vi "sendOpenLog.vi"(8 "error in (no error)":errorcluster, 11 "source":string) -> (0 "error out":errorcluster)   [LabVIEW 2017, in "loggingModule.lvlib"]
uses:
  loggingModule.lvlib
  Queue/TypeDefs/queueFGVState.ctl
  Queue/TypeDefs/message.ctl
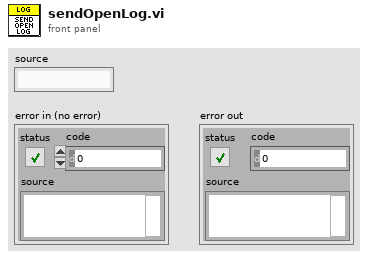
[diagram p1: front panel]
types:
  T1 = typedef "loggingModule.lvlib/message.ctl" = cluster{"calling module":string, "message":string, "data":variant}
  T2 = typedef "loggingModule.lvlib/queueFGVState.ctl" = enum16{"obtain", "enqueue low priority", "enqueue high priority", "dequeue", "release"}
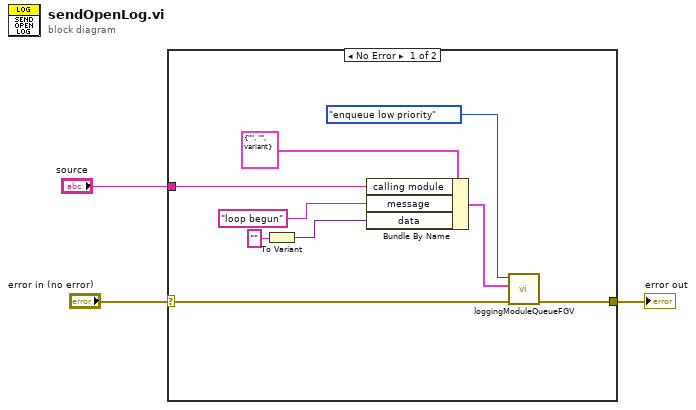
[diagram p0: block diagram]
diagram:
  n1 = case shown="No Error" "error in (no error)" {
    selector: "error in (no error)" -> [w4 w13]
    tunnel: [w12 w13] -> w3
    tunnel: "source" -> [w7 _]
    frame No Error {
      n2 = To Variant(anything="") -> (Variant=w10:variant)
      n3 = Bundle By Name(cluster=T1 {"calling module"="", "message"="", "data"=variant} ("message in"), "calling module"=w7, "message"="loop begun", "data"=w10) -> (w11:T1)
      n4 = call "loggingModuleQueueFGV.vi"("error in (no error)"=w4, "message in"=w11, "command"=queueFGVState."enqueue low priority") -> ("error out"=w12:errorcluster)  [unwired: 7 in, 1 out]
    }
    frame Error {
    }
  }
  "error out" <- w3
